vi "Main.vi"() -> ()   [LabVIEW 2021]
uses:
  Controls/Operation.ctl
  Controls/State Cluster.ctl
  Controls/Main Data Cluster.ctl
panel:
  out "error out":errorcluster
  in  "error in (no error)":errorcluster
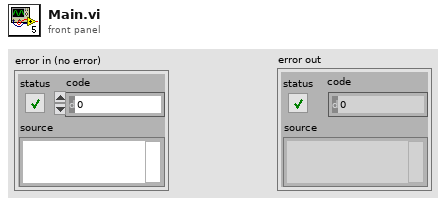
[diagram p1: front panel]
types:
  T1 = typedef "Main Data Cluster.ctl" = cluster{"user event out":refnum<user-event>}
  T2 = typedef "State Cluster.ctl" = cluster{"State":string, "Data":variant}
  T3 = typedef "Operation.ctl" = enum16{"Create", "Enqueue", "Enqueue N", "Enstack", "Dequeue", "Flush", "Release"}
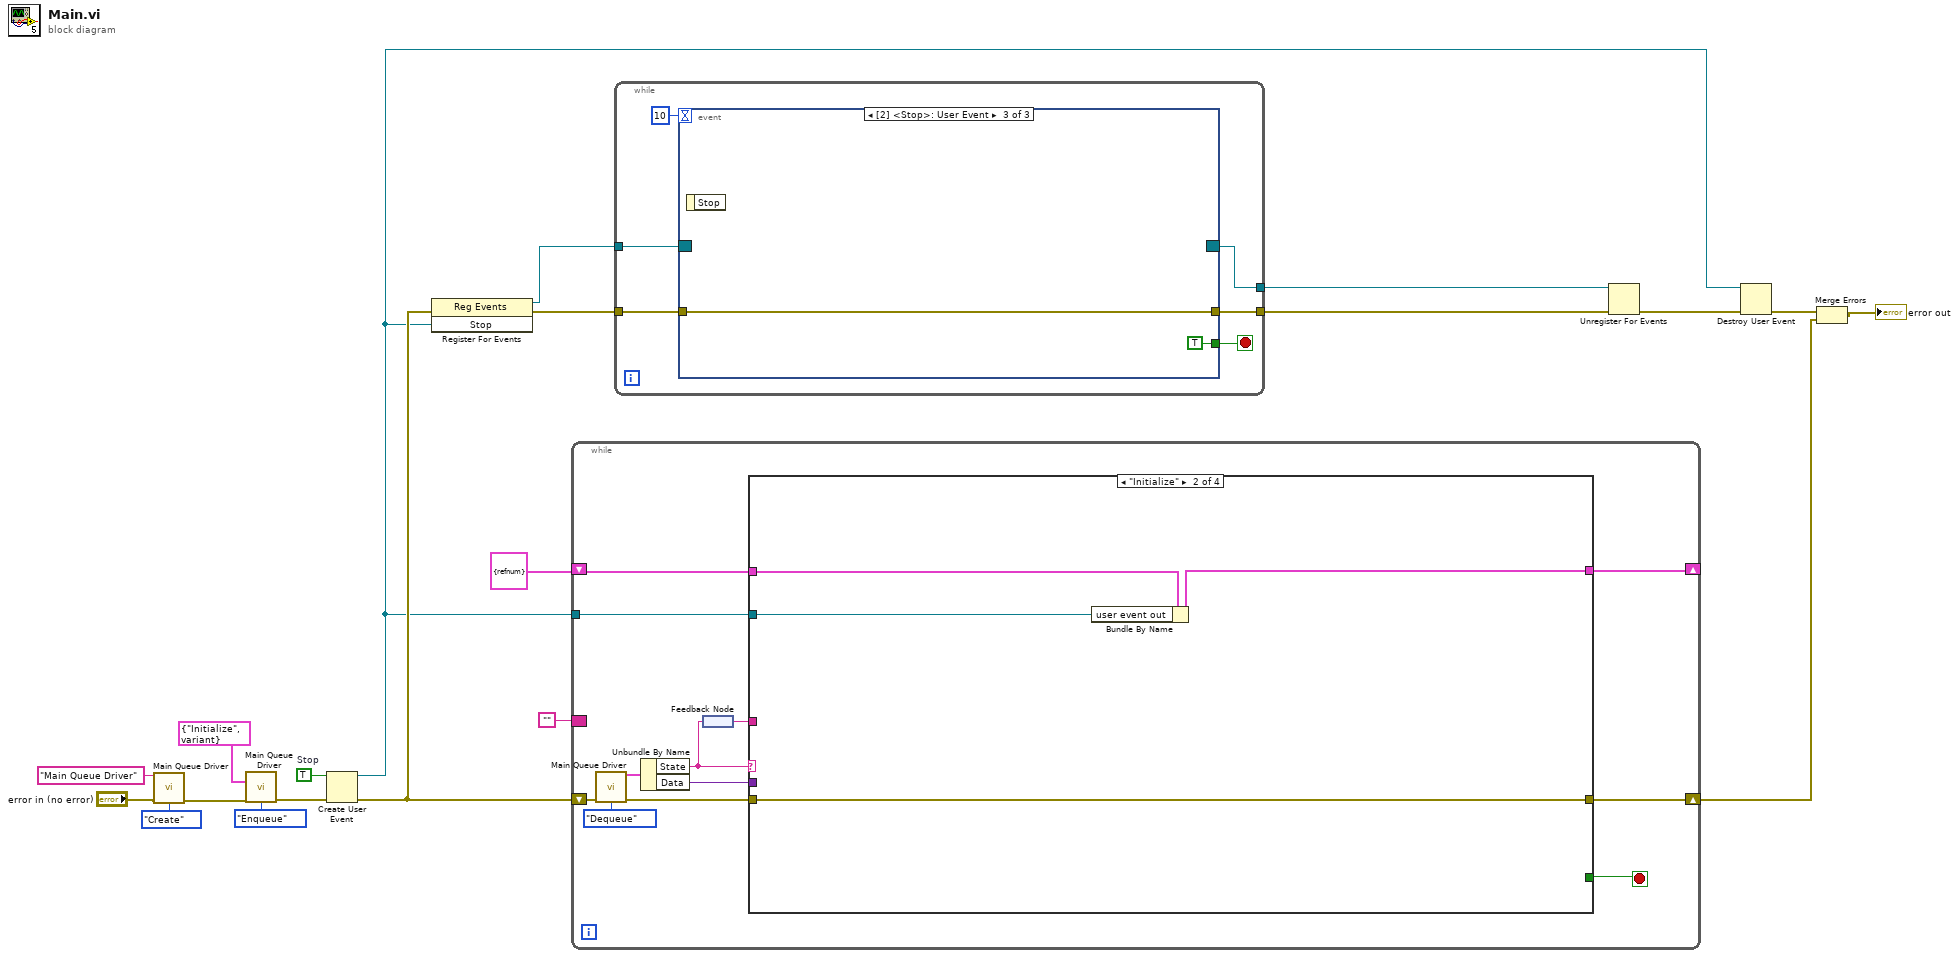
[diagram p0: block diagram]
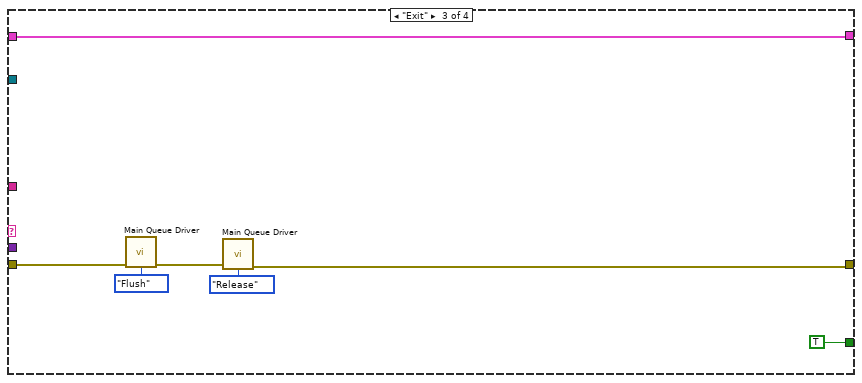
[diagram p3: hidden frame]
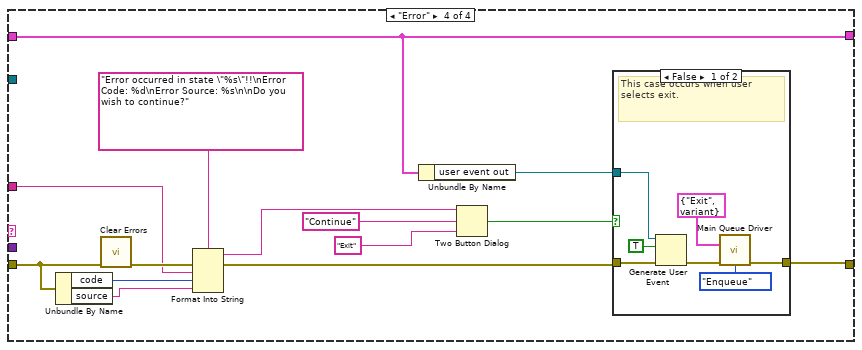
[diagram p4: hidden frame]
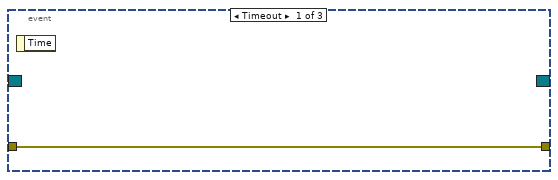
[diagram p6: hidden frame]
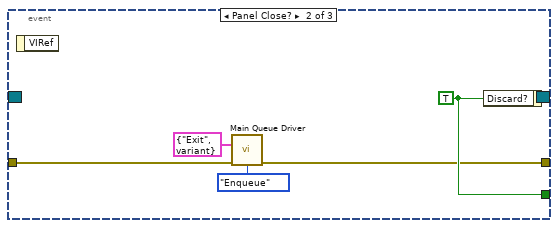
[diagram p7: hidden frame]
diagram:
  w13 = TRUE  # Stop
  n1 = call "Main Queue Driver.vi"("Queue Name"="Main Queue Driver", "error in (no error)"="error in (no error)", "Operations"=Operation."Create") -> ("error out"=w17:errorcluster)  [unwired: 11 in, 1 out]
  n2 = call "Main Queue Driver.vi"("State"=T2 {"State"="Initialize", "Data"=variant}, "error in (no error)"=w17, "Operations"=Operation."Enqueue") -> ("error out"=w14:errorcluster)  [unwired: 11 in, 1 out]
  n3 = Create User Event(user event datatype=w13, error in=w14) -> (user event=w1:refnum<user-event>, error out=w12:errorcluster)
  n4 = register-events(error in=w12, w1) -> (reference out=w10:refnum<event-registration>, error out=w11:errorcluster)  [unwired: 1 in]
  n5 = while {
    shift-right: [w26] -> w4
    shift-left: w12 -> [w31]
    border: "" -> [_]
    tunnel: w1 -> [w23]
    shift-right: [w22] -> _
    shift-left: T1 {"user event out"=refnum} -> [w24]
    stop <- w25 stop-if-true
    n6 = call "Main Queue Driver.vi"("error in (no error)"=w31, "Operations"=Operation."Dequeue") -> ("Dequeued Element"=w29:T2, "error out"=w30:errorcluster)  [unwired: 12 in]
    n7 = Unbundle By Name(w29) -> ("State"=w27:string, "Data"=w28:variant)
    n8 = feedback-in #1(w27) -> ()
    n9 = feedback #1() -> (w21:string)
    n10 = case shown="\"Initialize\"" w27 {
      tunnel: w30 -> [w34 w35 w44 w52]
      tunnel: w28 -> [_ _ _ _]
      tunnel: [w34 w35 w41 w49] -> w26
      tunnel: [_ _ TRUE _] -> w25
      tunnel: w24 -> [w33 w38 w39 w48]
      tunnel: w23 -> [_ w37 _ _]
      tunnel: [w33 w36 w39 w48] -> w22
      tunnel: w21 -> [_ _ _ w46]
      frame Default {
      }
      frame "Initialize" {
        n11 = Bundle By Name(cluster=w38, "user event out"=w37) -> (w36:T1)
      }
      frame "Exit" {
        n12 = call "Main Queue Driver.vi"("error in (no error)"=w44, "Operations"=Operation."Flush") -> ("error out"=w42:errorcluster)  [unwired: 12 in, 1 out]
        n13 = call "Main Queue Driver.vi"("error in (no error)"=w42, "Operations"=Operation."Release") -> ("error out"=w41:errorcluster)  [unwired: 12 in, 1 out]
      }
      frame "Error" {
        n14 = Unbundle By Name(w52) -> ("code"=w51:i32, "source"=w50:string)
        n15 = call <vilib>:"Clear Errors.vi"("error in (no error)"=w52) -> ("error out"=w59:errorcluster)  [unwired: 5 in, 1 out]
        n16 = Format Into String(format string="Error occurred in state \"%s\"!!\nError Code: %d\nError Source: %s\n\nDo you wish to continue?", error in=w59, w46, w51, w50) -> (resulting string=w57:string, error out=w54:errorcluster)  [unwired: 1 in]
        n17 = Unbundle By Name(w48) -> ("user event out"=w47:refnum<user-event>)
        n18 = Two Button Dialog(message=w57, 1:"Exit" ("F button name (\"Cancel\")"), 2:"Continue" ("T button name (\"OK\")")) -> (T button?=w53:bool)
        n19 = case shown="False" w53 {
          tunnel: w54 -> [w66 w67]
          tunnel: [w62 w67] -> w49
          tunnel: w47 -> [w64 _]
          frame False {
            # "This case occurs when user selects exit."
            n20 = Generate User Event(user event=w64, event data cluster=TRUE ("event data"), error in=w66) -> (error out=w63:errorcluster)  [unwired: 1 in, 1 out]
            n21 = call "Main Queue Driver.vi"("State"=T2 {"State"="Exit", "Data"=variant}, "error in (no error)"=w63, "Operations"=Operation."Enqueue") -> ("error out"=w62:errorcluster)  [unwired: 11 in, 1 out]
          }
          frame True {
            # "This case occurs when user selects to continue."
          }
        }
      }
    }
  }
  n22 = while {
    tunnel: w11 -> [w72]
    tunnel: w10 -> [w71]
    tunnel: [w70] -> w8
    tunnel: [w69] -> w7
    stop <- w68 stop-if-true
    n23 = event shown="[2] <Stop>: User Event" {
      selector: w71 -> [_ _ _]
      dyn-events: [_ _ _] -> w70
      timeout: 10 -> [_ _ _]
      tunnel: w72 -> [w74 w78 w81]
      tunnel: [w74 w77 w81] -> w69
      tunnel: [_ w79 TRUE ("Discard?")] -> w68
      event Timeout {
        n24 = event-data() -> ()  [unwired: 1 in, 1 out]
      }
      event Panel Close? {
        w79 = TRUE ("Discard?")
        n25 = event-data() -> ()  [unwired: 1 in, 1 out]
        n26 = call "Main Queue Driver.vi"("State"=T2 {"State"="Exit", "Data"=variant}, "error in (no error)"=w78, "Operations"=Operation."Enqueue") -> ("error out"=w77:errorcluster)  [unwired: 11 in, 1 out]
        n27 = event-data("Discard?"=w79) -> ()  [unwired: 1 in, 1 out]
      }
      event User Event {
        n28 = event-data() -> ()  [unwired: 1 in, 1 out]
      }
    }
  }
  n29 = Unregister For Events(event registration refnum=w8, error in=w7) -> (error out=w6:errorcluster)
  n30 = Destroy User Event(user event=w1, error in=w6) -> (error out=w5:errorcluster)
  n31 = Merge Errors(w5, w4) -> (→"error out":errorcluster)
